vi "PDash Add HL to Module.vi"(10 "Helper Loop Name":string, 11 "Module Info":T1) -> (0 "error out":errorcluster)   [LabVIEW 2020]
doc: "_____\nCreated using DQMH Event Scripter 7.1.0.1447."
uses:
  <vilib>/Delacor/Delacor QMH/Libraries/_Scripting Support/Module Info--cluster.ctl
  <vilib>/Delacor/Delacor QMH/Libraries/_Scripting Support/Module Type--enum.ctl
  PantherDashboard Scripting Hooks/Panther Dasboard Scripting Hooks.lvlib
  <vilib>/Delacor/Delacor QMH/Libraries/_Scripting Support/dqmh_lib_DQMH Scripting Support.lvlib
panel:
  in  "error in (no error)":errorcluster
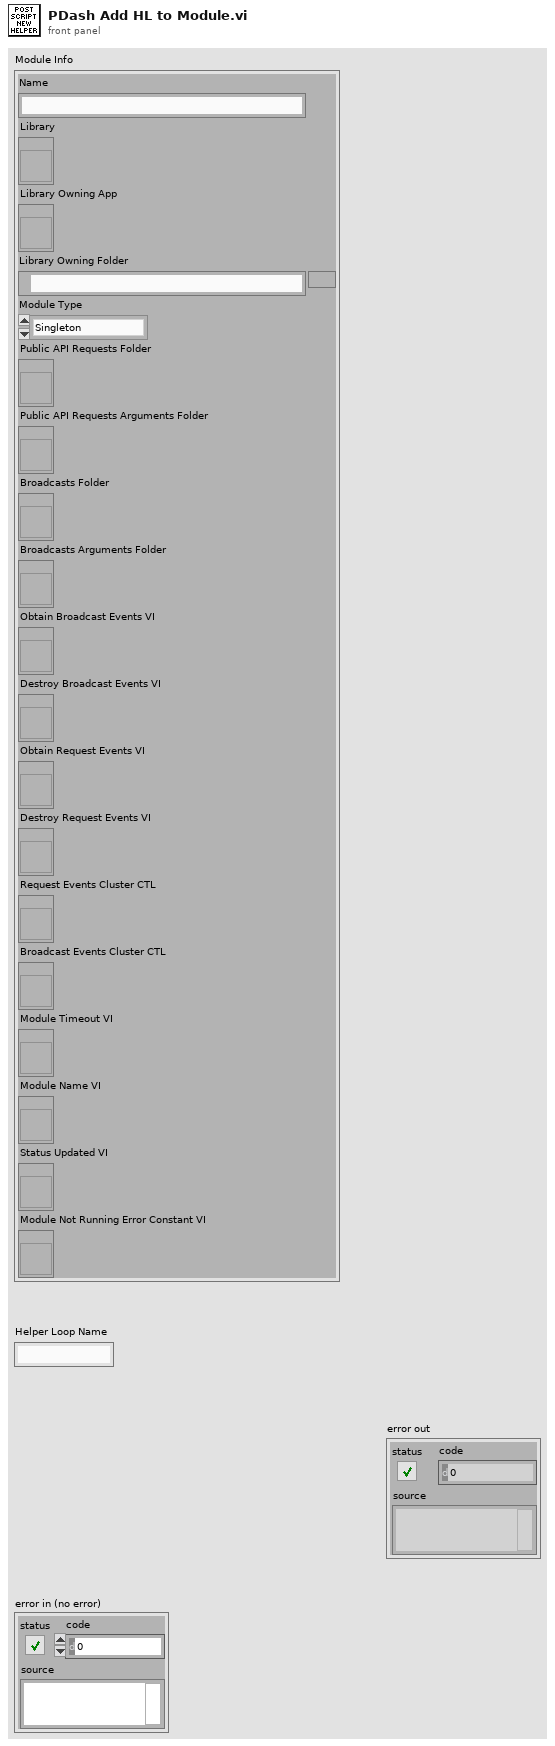
[diagram p1: front panel]
types:
  T1 = typedef "dqmh_lib_DQMH Scripting Support.lvlib/Module Info--cluster.ctl" = cluster{"Name":string, "Library":refnum<vi>, "Library Owning App":refnum<vi>, "Library Owning Folder":path, "Module Type":T2, "Public API Requests Folder":refnum<vi>, "Public API Requests Arguments Folder":refnum<vi>, "Broadcasts Folder":refnum<vi>, "Broadcasts Arguments Folder":refnum<vi>, "Obtain Broadcast Events VI":refnum<vi>, "Destroy Broadcast Events VI":refnum<vi>, "Obtain Request Events VI":refnum<vi>, "Destroy Request Events VI":refnum<vi>, "Request Events Cluster CTL":refnum<vi>, "Broadcast Events Cluster CTL":refnum<vi>, "Module Timeout VI":refnum<vi>, "Module Name VI":refnum<vi>, "Status Updated VI":refnum<vi>, "Module Not Running Error Constant VI":refnum<vi>}
  T2 = typedef "dqmh_lib_DQMH Scripting Support.lvlib/Module Type--enum.ctl" = enum16{"Singleton", "Cloneable"}
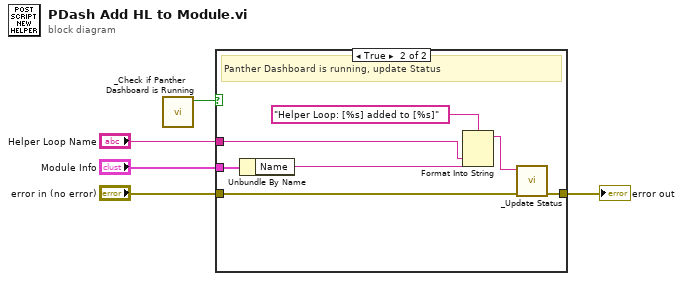
[diagram p0: block diagram]
diagram:
  n1 = call "_Check if Panther Dashboard is Running.vi"() -> ("Panther Dashboard is Running?"=w1:bool)  [unwired: 10 in, 1 out]
  n2 = case shown="True" w1 {
    tunnel: [w6 w12] -> w5
    tunnel: "error in (no error)" -> [w6 w13]
    tunnel: "Helper Loop Name" -> [_ w8]
    tunnel: "Module Info" -> [_ w10]
    frame False {
    }
    frame True {
      # "Panther Dashboard is running, update Status"
      n3 = Unbundle By Name(w10) -> ("Name"=w9:string)
      n4 = Format Into String(format string="Helper Loop: [%s] added to [%s]", w8, w9) -> (resulting string=w7:string)  [unwired: 2 in, 1 out]
      n5 = call "_Update Status.vi"("error in"=w13, "Status"=w7) -> ("error out"=w12:errorcluster)  [unwired: 9 in]
    }
  }
  "error out" <- w5
